vi "Write NCh NSamp (I32).vi"(5 "timestamps":timestamp[](array[numeric]), 7 "index_channel":u32, 8 "error in":errorcluster, 9 "data":i32[][](array[numeric]), 10 "channels":u32[](array[numeric]), 11 "writer":u64) -> (0 "error out":errorcluster, 3 "writer out":u64)   [LabVIEW 2026, in "synnax_clib.lvlib"]
uses:
  synnax_clib.lvlib
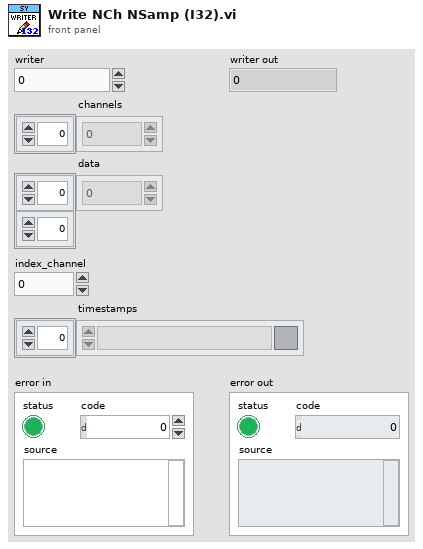
[diagram p1: front panel]
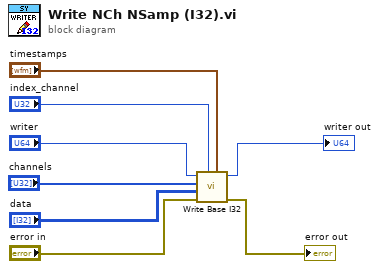
[diagram p0: block diagram]
diagram:
  n1 = call "Write Base I32.vi"("timestamps"="timestamps", "index_channel"="index_channel", "error in"="error in", "data"="data", "channels"="channels", "writer"="writer") -> ("error out"=→"error out":errorcluster, "writer out"=→"writer out":u64)  [unwired: 4 in]
